vi "Recurrence for Rational Interpolation.vi"(1 "R(i+1)...(i+m)":dbl format="%0.2f", 2 "x":dbl format="%0.2f", 3 "R(i+1)...(i+m-1)":dbl format="%0.2f", 4 "R(i)...(i+m-1)":dbl format="%0.2f", 5 "x2":dbl format="%0.2f", 6 "x1":dbl format="%0.2f") -> (0 "Ri(i+1)...(i+m)":dbl format="%0.2f")   [LabVIEW 2020, in "NI_PtbyPt.lvlib"]
uses:
  <vilib>/ptbypt/NI_PtbyPt.lvlib
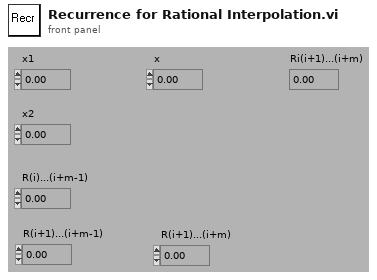
[diagram p1: front panel]
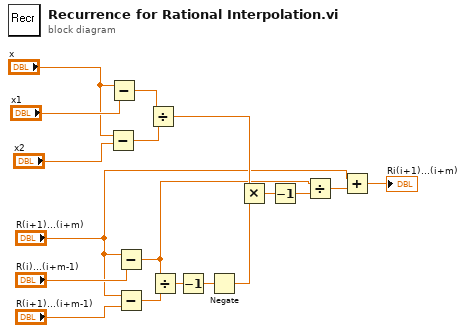
[diagram p0: block diagram]
diagram:
  n1 = Subtract(x="x", y="x2") -> (x-y=w9:dbl)
  n2 = Subtract(x="x", y="x1") -> (x-y=w10:dbl)
  n3 = Subtract(x="R(i+1)...(i+m)", y="R(i)...(i+m-1)") -> (x-y=w4:dbl)
  n4 = Subtract(x="R(i+1)...(i+m)", y="R(i+1)...(i+m-1)") -> (x-y=w16:dbl)
  n5 = Divide(x=w10, y=w9) -> (x/y=w8:dbl)
  n6 = Divide(x=w4, y=w16) -> (x/y=w15:dbl)
  n7 = Decrement(x=w15) -> (x-1=w14:dbl)
  n8 = Negate(x=w14) -> (-x=w7:dbl)
  n9 = Multiply(x=w8, y=w7) -> (x*y=w6:dbl)
  n10 = Decrement(x=w6) -> (x-1=w5:dbl)
  n11 = Divide(x=w4, y=w5) -> (x/y=w3:dbl)
  n12 = Add(x="R(i+1)...(i+m)", y=w3) -> (x+y=→"Ri(i+1)...(i+m)":dbl)
